vi "Throw -8718 error.vi"(8 "error in (no error)":errorcluster, 9 "path":path, 10 "Custom device name":string, 11 "Error":bool) -> (0 "error out":errorcluster)   [LabVIEW 2020, in "Engine Simulation Toolkit System Explorer.lvlib"]
uses:
  Engine Simulation Toolkit System Explorer.lvlib
  <vilib>/Utility/error.llb/Error Cluster From Error Code.vi
  <vilib>/ErrorRing/Error Ring.xnode
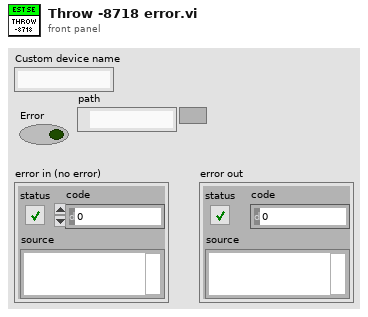
[diagram p1: front panel]
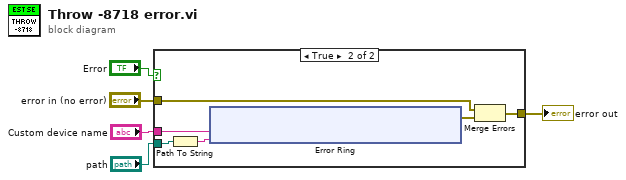
[diagram p0: block diagram]
diagram:
  n1 = case shown="True" "Error" {
    tunnel: "error in (no error)" -> [w6 w12]
    tunnel: "Custom device name" -> [_ w10]
    tunnel: [w6 w9] -> w5
    tunnel: "path" -> [_ w8]
    frame False {
    }
    frame True {
      n2 = Path To String(path=w8) -> (string=w7:string)
      n3 = xnode "Error Ring"("parameter 0"=w10, "parameter 1"=w7) -> ("error out"=w11:errorcluster)
      n4 = Merge Errors(w12, w11) -> (w9:errorcluster)
    }
  }
  "error out" <- w5
